vi "MultiDimensionalArrays.vi"(6 "Array":cluster{"Numeric":dbl, "Array":dbl[][]}[][](array[cluster])=[[{"Numeric"=111.0, "Array"=[[11.0, 21.0], [31.0, 41.0]]}, {"Numeric"=222.0, "Array"=[[12.0, 22.0], [32.0, 42.0]]}], [{"Numeric"=333.0, "Array"=[[13.0, 23.0], [33.0, 43.0]]}, {"Numeric"=444.0, "Array"=[[14.0, 24.0], [34.0, 44.0]]}]], 7 "Numeric Array":dbl[][](array[numeric])=[[1.0, 2.0, 3.0], [4.0, 5.0, 6.0], [7.0, 8.0, 9.0]], 8 "Cluster":T1={"Numeric Array"=[[[11.0, 21.0, 31.0], [41.0, 51.0, 61.0], [71.0, 81.0, 91.0]], [[55.0, 0.0, 0.0], [0.0, 88.0, 0.0], [0.0, 0.0, 99.0]]], "String Array"=[["aaa", "bbb"], ["ccc", "ddd"]]}, 9 "String Array":string[][](array[string])=[["AAAAA", "BBBBB"], ["CCCCC", "DDDDD"]], 10 "Numeric Array 3D 2":dbl[][][][](array[numeric])=[[[[111.0, 222.0], [333.0, 444.0], [555.0, 777.0]], [[888.0, 999.0], [1000.0, 1110.0], [2220.0, 3330.0]]], [[[1234.0, 678.0], [12378.0, 1122.0], [3344.0, 5577.0]], [[12.0, 12.0], [12.0, 12.0], [12.0, 12.0]]]], 11 "Numeric Array 3D":dbl[][][](array[numeric])=[[[111.0, 222.0], [333.0, 444.0], [555.0, 777.0], [1257.0, 7543.0]], [[888.0, 999.0], [1000.0, 1110.0], [2220.0, 3330.0], [12.0, 12.0]]]) -> ()   [LabVIEW 2012]
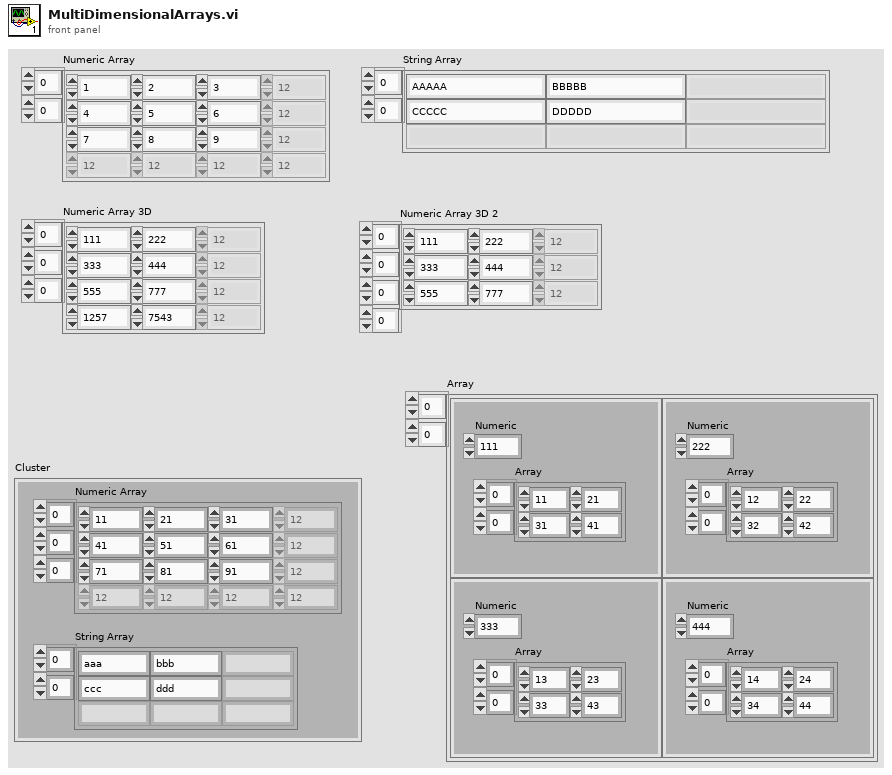
[diagram p1: front panel]
types:
  T1 = cluster{"Numeric Array":dbl[][][], "String Array":string[][]}
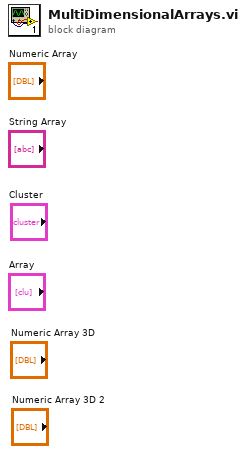
[diagram p0: block diagram]
diagram:
